vi "Sensors_to_csv.vi"() -> ()   [LabVIEW 2020]
uses:
  <vilib>/express/express analysis/Spectral/Block/exnSpectralBlock spectral measurements peak poly.vi
  <vilib>/express/express analysis/Spectral/Block/exnSpectralBlock spectral measurements peak DDT.vi
  <vilib>/express/express analysis/Spectral/XNode/ExpressSpectralMeasurementsBlockNode.xnode
panel:
  in  "Current":dbl(slide) scale=2.5..2.6
  out "Vibration Peak":dbl
  out "fft-peak":dbl
  out "data 2":dynamicdata(graph) caption="Sensor Output"
  out "Sensor output":dbl
  out "Current":dbl
  out "Gauge":dbl(knob) scale=0.0..5.0
  out "Temperature":dbl
  out "Thermometer":dbl(slide) scale=0.0..100.0
  in  "System stop":bool
  out "RPM":dbl
  out "FFT":dynamicdata(graph)
  out "Time Domain":dynamicdata(graph)
  out "Time Domain":dynamicdata(graph)
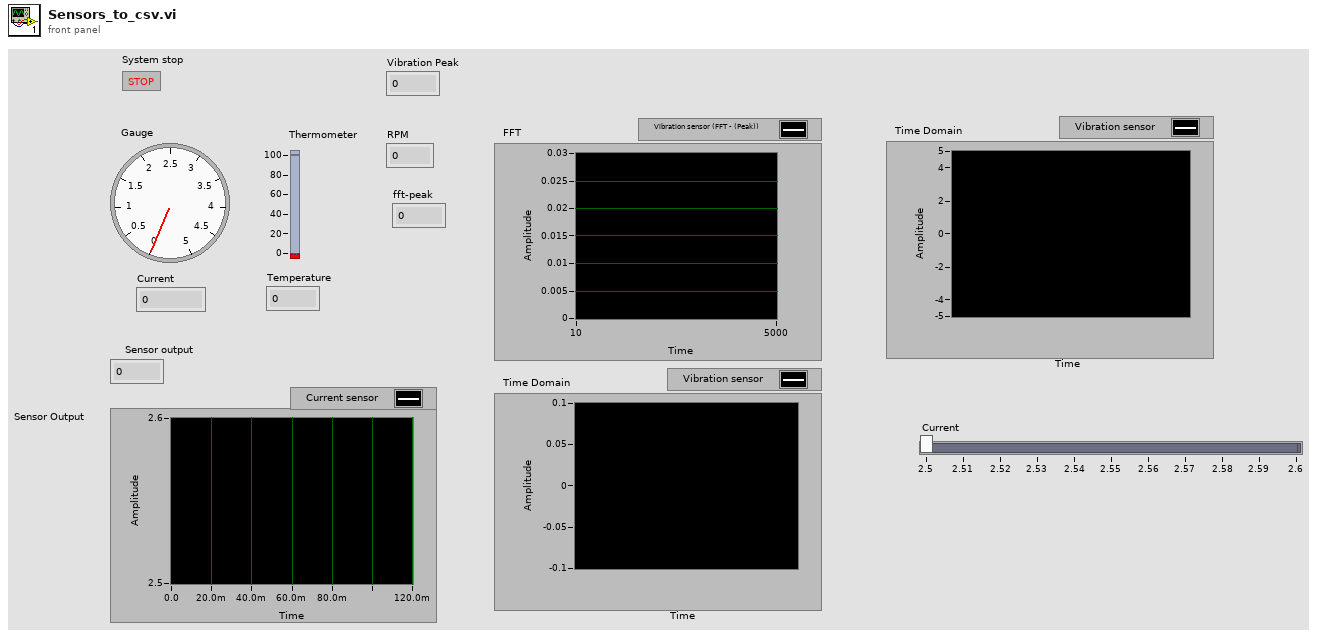
[diagram p1: front panel]
types:
  T1 = enum16{"open", "replace", "create", "open or create", "replace or create", "replace or create with confirmation"}
  T2 = cluster{"averaging mode":u16, "weighting mode":u16, "number of averages":u32}
  T3 = cluster{"dB On (F)":bool, "unwrap phase (F)":bool, "convert to degree (F)":bool}
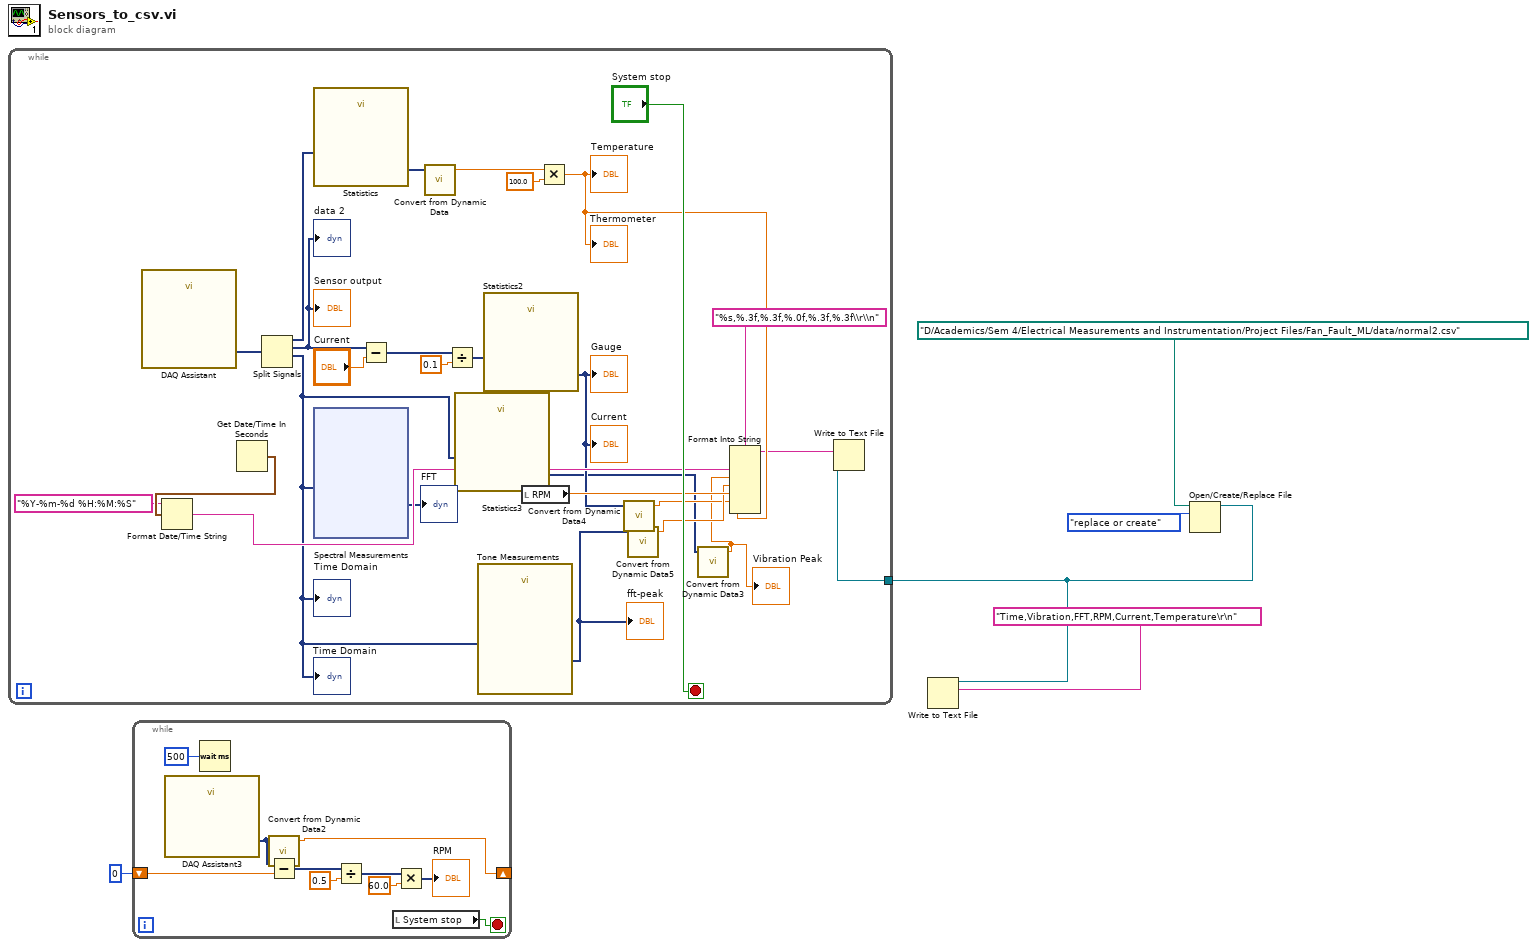
[diagram p0: block diagram]
diagram:
  n1 = while {
    shift-right: [w13] -> _
    shift-left: 0 -> [w14]
    stop <- w6 stop-if-true
    n2 = call "DAQ Assistant3"() -> ("data"=w7:dynamicdata)  [unwired: 16 in, 3 out]
    n3 = Wait (ms)(milliseconds to wait=u32 500) -> ()  [unwired: 1 out]
    n4 = call "Convert from Dynamic Data2"("Dynamic Data Type"=w7) -> ("Scalar"=w13:dbl)  [unwired: 3 in]
    n5 = Subtract(x=w7, y=w14) -> (x-y=w12:dynamicdata)
    n6 = Divide(x=w12, y=0.5) -> (x/y=w11:dynamicdata)
    n7 = local read "System stop"() -> (w6:bool)
    n8 = Multiply(x=w11, y=60.0) -> (x*y=→"RPM":dynamicdata)
  }
  n9 = Open/Create/Replace File(file path (use dialog)=path "D:/Academics/Sem 4/Electrical Measurements and Instrumentation/Project Files/Fan_Fault_ML/data/normal2.csv", operation (0:open)=T1."replace or create") -> (refnum out=w1:refnum<file>)  [unwired: 4 in, 2 out]
  n10 = while {
    tunnel: w1 -> [w21]
    stop <- "System stop" stop-if-true
    n11 = call "DAQ Assistant"() -> ("data"=w36:dynamicdata)  [unwired: 16 in, 3 out]
    n12 = Get Date/Time In Seconds() -> (seconds since 1Jan1904=w32:timestamp)
    n13 = Format Date/Time String(time format string (%c)="%Y-%m-%d %H:%M:%S", seconds (now)=w32) -> (date/time string=w29:string)  [unwired: 1 in]
    n14 = Split Signals(w36) -> (w33:dynamicdata, w35:dynamicdata, w19:dynamicdata)  [unwired: 4 in, 1 out]
    "Time Domain" <- w19
    "Time Domain" <- w19
    "Sensor output" <- w35
    "data 2" <- w35
    n15 = call "Statistics"("Signals"=w33) -> ("Arithmetic Mean"=w41:dynamicdata)  [unwired: 25 in, 1 out]
    n16 = xnode "Spectral Measurements"("Signals"=w19) -> ("FFT - (Peak)"=→"FFT":dynamicdata)  [unwired: 1 in, 2 out]
    n17 = Subtract(x=w35, y="Current") -> (x-y=w38:dynamicdata)
    n18 = call "Convert from Dynamic Data"("Dynamic Data Type"=w41) -> ("Scalar"=w40:dbl)  [unwired: 3 in]
    n19 = Divide(x=w38, y=0.1) -> (x/y=w34:dynamicdata)
    n20 = call "Statistics3"("Signals"=w19) -> ("Maximum"=w18:dynamicdata)  [unwired: 25 in, 1 out]
    n21 = call "Tone Measurements"("Signals"=w19) -> ("Frequency"=w20:dynamicdata)  [unwired: 8 in, 2 out]
    "fft-peak" <- w20
    n22 = call "Statistics2"("Signals"=w34) -> ("Arithmetic Mean"=w25:dynamicdata)  [unwired: 25 in, 1 out]
    "Gauge" <- w25
    "Current" <- w25
    n23 = local read "RPM"() -> (w28:dbl)
    n24 = Multiply(x=w40, y=100.0) -> (x*y=w27:dbl)
    "Thermometer" <- w27
    "Temperature" <- w27
    n25 = call "Convert from Dynamic Data4"("Dynamic Data Type"=w25) -> ("Scalar"=w22:dbl)  [unwired: 3 in]
    n26 = call "Convert from Dynamic Data5"("Dynamic Data Type"=w20) -> ("Scalar"=w24:dbl)  [unwired: 3 in]
    n27 = call "Convert from Dynamic Data3"("Dynamic Data Type"=w18) -> ("Scalar"=w17:dbl)  [unwired: 3 in]
    "Vibration Peak" <- w17
    n28 = Format Into String(format string="%s,%.3f,%.3f,%.0f,%.3f,%.3f\\r\\n", w29, w17, w24, w28, w22, w27) -> (resulting string=w26:string)  [unwired: 2 in, 1 out]
    n29 = Write to Text File(file (use dialog)=w21, text=w26) -> ()  [unwired: 2 in, 3 out]
  }
  n30 = Write to Text File(file (use dialog)=w1, text="Time,Vibration,FFT,RPM,Current,Temperature\r\n") -> ()  [unwired: 2 in, 3 out]
